vi "Main.vi"() -> ()   [LabVIEW 2012]
uses:
  Car Wash Controller/Car Wash Controller/Load App.vi
  Car Wash Controller/Car Wash Controller/Car Wash Controller.lvclass
panel:
  out "Waiting Lights":T1
  out "Current action:":string
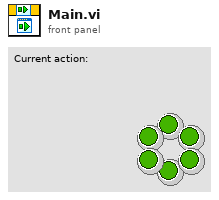
[diagram p1: front panel]
types:
  T1 = cluster{"DNL_wait 1":bool, "DNL_wait 1":bool, "DNL_wait 1":bool, "DNL_wait 1":bool, "DNL_wait 1":bool, "DNL_wait 1":bool}
  T2 = cluster{"[0]":bool, "[1]":bool, "[2]":bool, "[3]":bool, "[4]":bool, "[5]":bool}
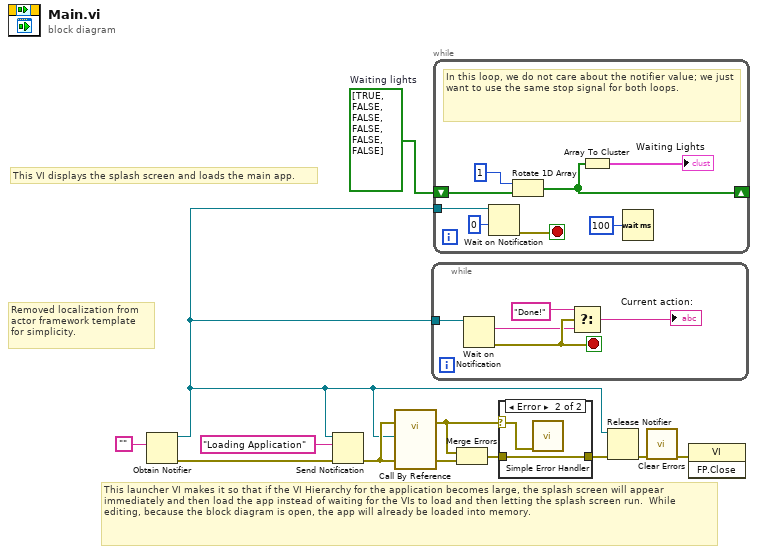
[diagram p0: block diagram]
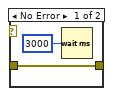
[diagram p2: hidden frame]
diagram:
  w6 = bool[] [TRUE, FALSE, FALSE, FALSE, FALSE, FALSE]  # Waiting lights
  # "This VI displays the splash screen and loads the main app."
  # "Removed localization from\nactor framework template \nfor simplicity."
  # "This launcher VI makes it so that if the VI Hierarchy for the application becomes large, the splash screen will appear immediately and then load the app instead of waiting for the VIs to load and then letting the splash screen run.  While editing, because the block diagram is open, the app will already be loaded into memory."
  n1 = Obtain Notifier(notification data type="") -> (notifier out=w8:refnum<notifier>, error out=w4:errorcluster)  [unwired: 3 in, 1 out]
  n2 = Send Notification(notification="Loading Application", notifier=w8, error in (no error)=w4) -> (error out=w9:errorcluster)  [unwired: 1 out]
  n3 = call-by-ref "?"(error in=w9, 8:"error in (no error)"=w9, "Status Notifier"=w8) -> (error out=w1:errorcluster, 0:"error out"=w12:errorcluster)  [unwired: 10 in, 1 out]
  n4 = while {
    tunnel: w8 -> [w17]
    stop <- w16 stop-if-true
    n5 = Wait on Notification(notifier=w17) -> (notification=w14:string, error out=w16:errorcluster)  [unwired: 3 in, 2 out]
    n6 = Select(t="Done!" ("notification"), s=w16, f=w14) -> (s? t:f=→"Current action:":string)
  }
  n7 = while {
    shift-right: [w19] -> _
    shift-left: w6 -> [w21]
    tunnel: w8 -> [w23]
    stop <- w25 stop-if-true
    # "In this loop, we do not care about the notifier value; we just want to use the same stop signal for both loops."
    n8 = Wait on Notification(notifier=w23, timeout in ms (-1)=0) -> (error out=w25:errorcluster)  [unwired: 2 in, 3 out]
    n9 = Rotate 1D Array(1:w21, 2:1 ("n")) -> (0:w19:bool[])
    n10 = Array To Cluster(array=w19) -> (cluster=→"Waiting Lights":T2)
    n11 = Wait (ms)(milliseconds to wait=u32 100) -> ()  [unwired: 1 out]
  }
  n12 = Merge Errors(w1, w12) -> (w2:errorcluster)
  n13 = case shown="Error" w1 {
    tunnel: [w27 w28] -> w3
    tunnel: w2 -> [w27 w28]
    selector: w1 -> [_ w29]
    frame No Error {
      n14 = Wait (ms)(milliseconds to wait=u32 3000) -> ()  [unwired: 1 out]
    }
    frame Error {
      n15 = call <vilib>:"Simple Error Handler.vi"("error in (no error)"=w29) -> ()  [unwired: 4 in, 5 out]
    }
  }
  n16 = Release Notifier(notifier=w8, error in (no error)=w3) -> (error out=w11:errorcluster)  [unwired: 1 in, 2 out]
  n17 = call <vilib>:"Clear Errors.vi"("error in (no error)"=w11) -> ("error out"=w5:errorcluster)  [unwired: 5 in, 1 out]
  n18 = invoke class="VI" method="FP.Close"(error in=w5) -> ()  [unwired: 2 in, 3 out]
